vi "WS1050_36 DUT CV Curve SData Ver1.0.vi"(0 "TMN DC\\CAP Data Log File Path":path=path "C:/temp", 1 "Lot#":string="WS1050", 2 "Total Delta C1(pF)":string[](array[string]), 3 "VSA_V1":string[][](array[string]), 4 "Wafer#":string="T7", 5 "File Name":string="Test Data", 6 "Total Delta C2(pF)":string[](array[string]), 7 "error in":errorcluster, 8 "TP/Comment":T1={"Test Program"="Multi Socket", "Comment"="HD_Cycling", "DVA"="", "EFUSE CAL"="", "CP HD/CYC"="", "VDD"="", "Duty Cycle"="", "V_Test(V)"="", "V_VPI(V)"="", "Freq(Hz)"="", "Board#"=""}, 9 "EFuse":string[](array[string])=["NC", "NC", "NC", "NC", "NC", "NC", "NC", "NC", "NC", "NC", "NC", "NC", "NC", "NC", "NC", "NC", "NC", "NC", "NC", "NC", "NC", "NC", "NC", "NC", "NC", "NC", "NC", "NC", "NC", "NC", "NC", "NC", "NC", "NC", "NC", "NC"], 10 "Data Output C3":string[][](table), 11 "Temperature":string="WS1033", 12 "VSA_V2":string[][](array[string]), 13 "VPI C3":string[][](array[string]), 14 "Data Output C1":string[][](table), 15 "VPI C2":string[][](array[string]), 16 "SN":string[](array[string])=["1", "2", "3", "4", "5", "6", "7", "8", "9", "10", "11", "12", "13", "14", "15", "16", "17", "18", "19", "20", "21", "22", "23", "24", "25", "26", "27", "28", "29", "30", "31", "32", "33", "34", "35", "36"], 17 "R/W Status":string[](array[string])=["PASS", "PASS", "PASS", "PASS", "PASS", "PASS", "PASS", "PASS", "PASS", "PASS", "PASS", "PASS", "PASS", "PASS", "PASS", "PASS", "PASS", "PASS", "PASS", "PASS", "PASS", "PASS", "PASS", "PASS", "PASS", "PASS", "PASS", "PASS", "PASS", "PASS", "PASS", "PASS", "PASS", "PASS", "PASS", "PASS"], 18 "Cap Header":string[](array[string]), 20 "HD/Cycles Completed":string="Test Data", 21 "Data Output C2":string[][](table), 23 "VSA_V3":string[][](array[string]), 24 "Current":string[](array[string]), 25 "VPI C1":string[][](array[string]), 26 "Total Delta C3(pF)":string[](array[string])) -> (27 "error out":errorcluster)   [LabVIEW 2012]
panel:
  in  "Bin":string[](array[string])=["NC", "NC", "NC", "NC", "NC", "NC", "NC", "NC", "NC", "NC", "NC", "NC", "NC", "NC", "NC", "NC", "NC", "NC", "NC", "NC", "NC", "NC", "NC", "NC", "NC", "NC", "NC", "NC", "NC", "NC", "NC", "NC", "NC", "NC", "NC", "NC"]
  # "*********** Do Not Remove ***********\nCompany:  WiSpry Inc\n20 Fairbanks Ste 198 Irvine CA 92618\n\nAuthor:  Andy V Tran\nCreated:  09/17/2014\nLabVIEW 2012 Suite\nTP:  Multi-Socket Save Data ver1.0\n*****************************************"
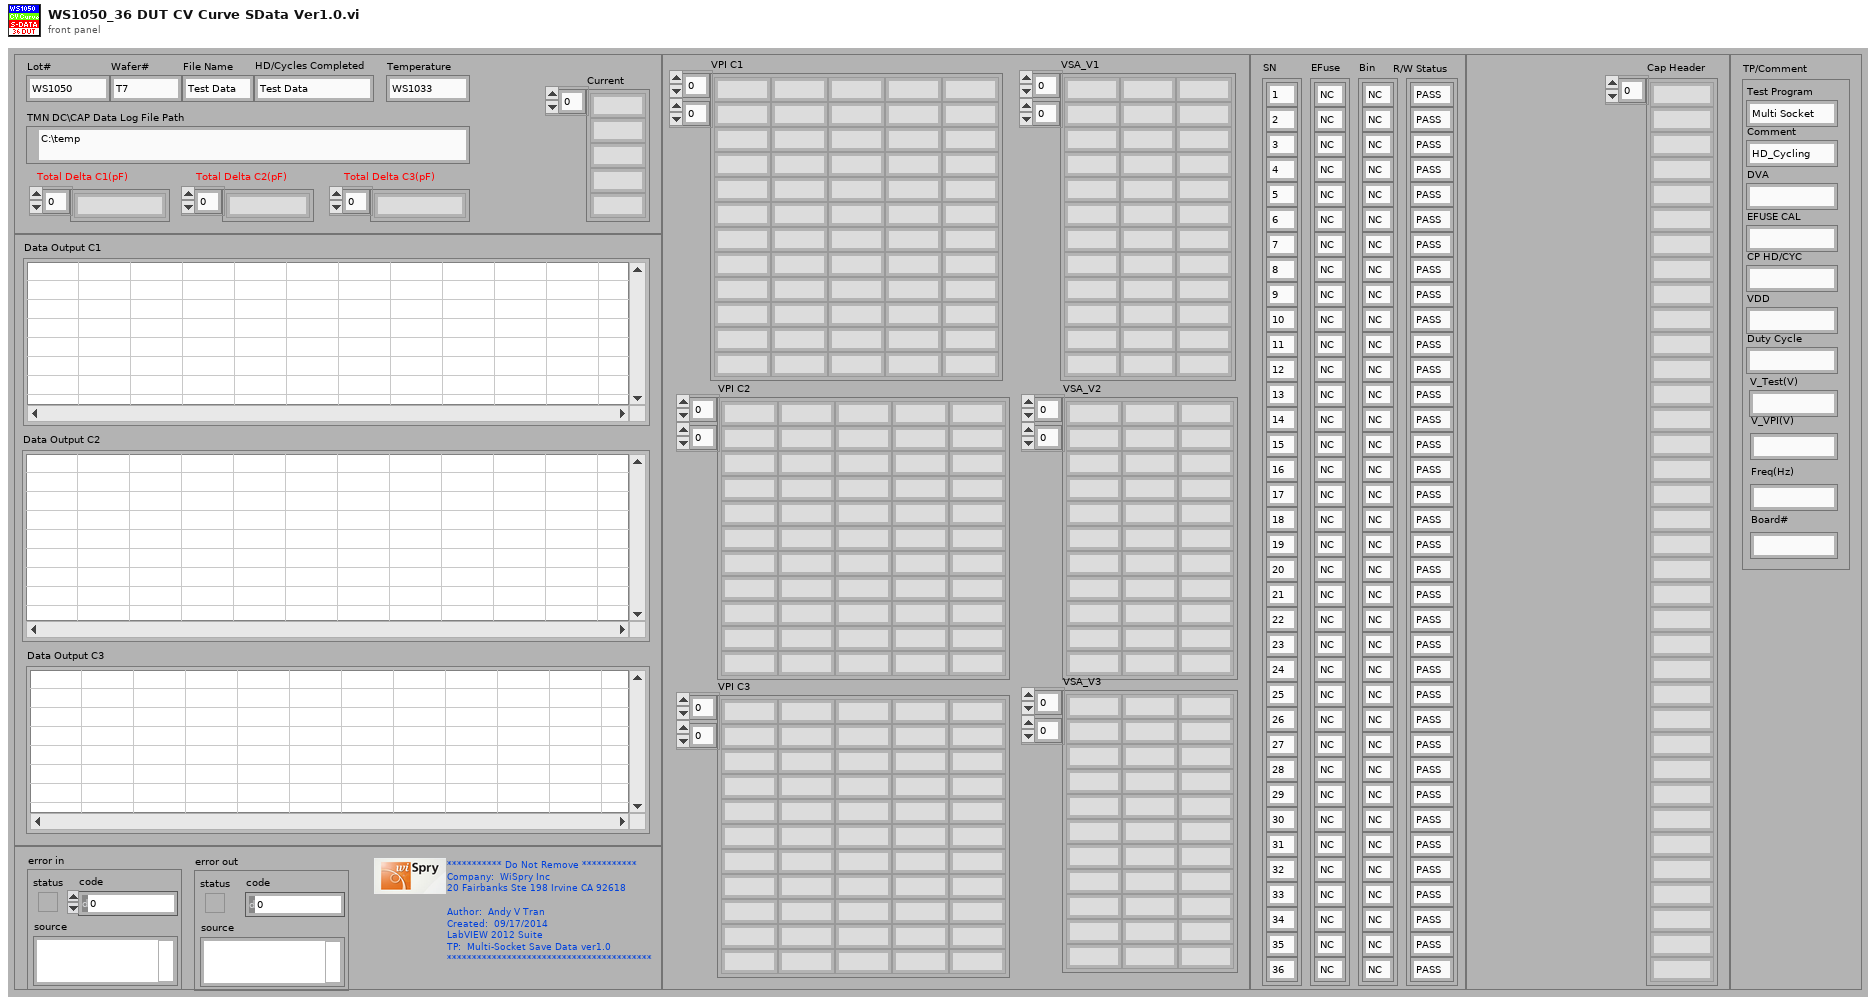
[diagram p1: front panel]
types:
  T1 = cluster{"Test Program":string, "Comment":string, "DVA":string, "EFUSE CAL":string, "CP HD/CYC":string, "VDD":string, "Duty Cycle":string, "V_Test(V)":string, "V_VPI(V)":string, "Freq(Hz)":string, "Board#":string}
  T2 = enum16{"open", "replace", "create", "open or create", "replace or create", "replace or create with confirmation"}
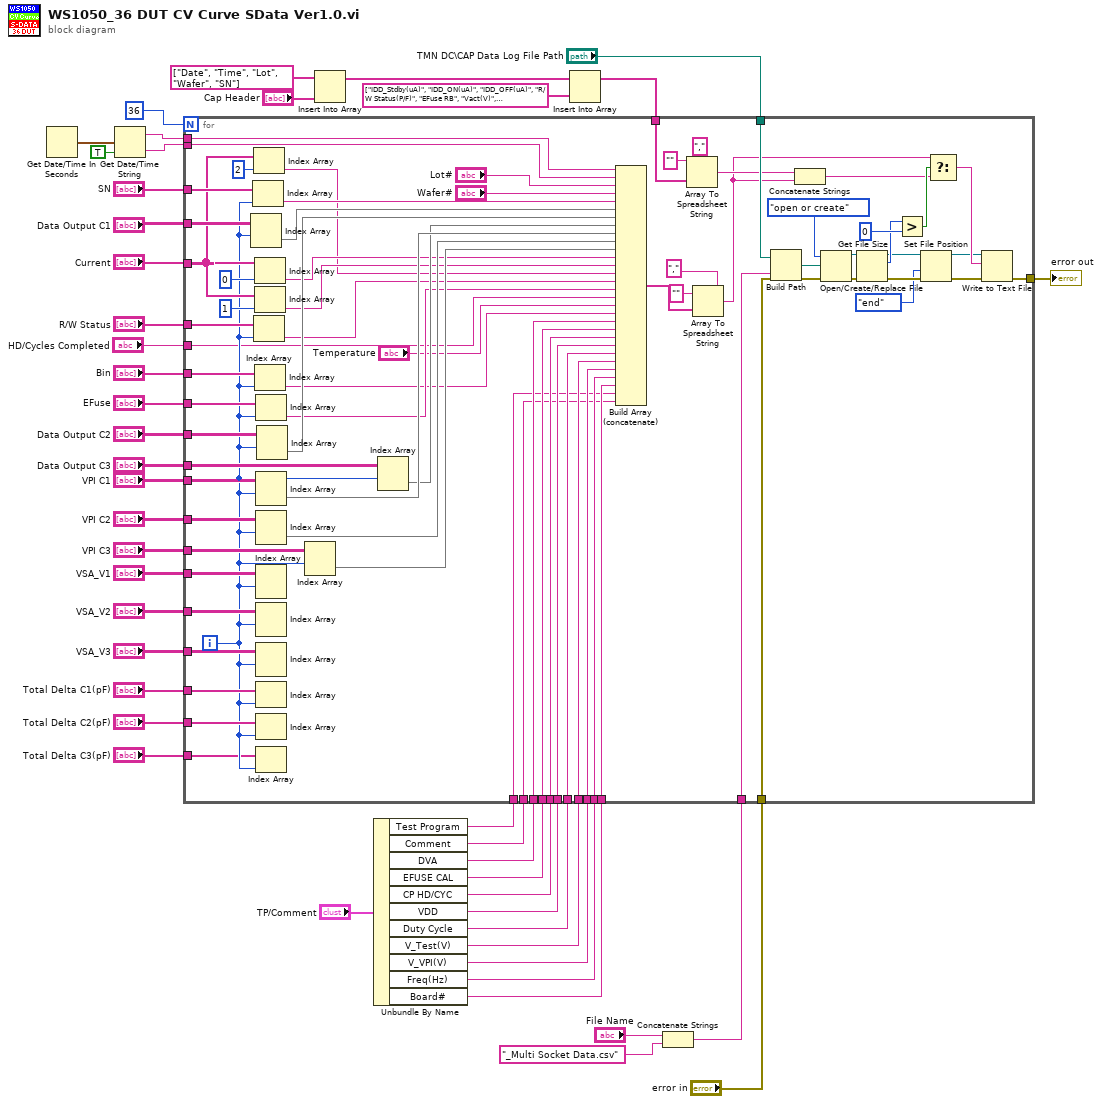
[diagram p0: block diagram]
diagram:
  n1 = Get Date/Time In Seconds() -> (seconds since 1Jan1904=w25:timestamp)
  n2 = Get Date/Time String(seconds (now)=w25, want seconds? (F)=TRUE) -> (date string=w33:string, time string=w34:string)  [unwired: 1 in]
  n3 = Insert Into Array(array=string[] ["Date", "Time", "Lot", "Wafer", "SN"], new element="Cap Header") -> (w12:string[])  [unwired: 1 in]
  n4 = Unbundle By Name("TP/Comment") -> ("Test Program"=w38:string, "Comment"=w37:string, "DVA"=w11:string, "EFUSE CAL"=w10:string, "CP HD/CYC"=w9:string, "VDD"=w8:string, "Duty Cycle"=w7:string, "V_Test(V)"=w6:string, "V_VPI(V)"=w5:string, "Freq(Hz)"=w3:string, "Board#"=w2:string)
  n5 = Insert Into Array(array=w12, new element=string[] ["IDD_Stdby(uA)", "IDD_ON(uA)", "IDD_OFF(uA)", "R/W Status(P/F)", "EFuse RB", "Vact(V)", "Temperature", "Bin", "DVA ON/OFF", "CAL ON/OFF", "CP_Sweep(V)", "VDD", "Duty Cycle(%)", "V_Test(V)", "V_VPI(V)", "Freq(Hz)", "Board", "Test Program", "Comment"]) -> (w16:string[])  [unwired: 1 in]
  n6 = Concatenate Strings("File Name", "_Multi Socket Data.csv" ("string")) -> (w41:string)
  n7 = for {
    N: 36 -> [_]
    tunnel: "TMN DC\\CAP Data Log File Path" -> [w123]
    tunnel: w16 -> [w122]
    tunnel: "error in" -> [w83]
    tunnel: w41 -> [w121]
    tunnel: [w99] -> w40
    tunnel: "SN" -> [w98]
    tunnel: "Current" -> [w90]
    tunnel: w38 -> [w48]
    tunnel: w37 -> [w47]
    tunnel: "Bin" -> [w97]
    tunnel: "R/W Status" -> [w96]
    tunnel: w34 -> [w73]
    tunnel: w33 -> [w72]
    tunnel: "Data Output C1" -> [w95]
    tunnel: "Data Output C2" -> [w94]
    tunnel: "VPI C1" -> [w89]
    tunnel: "VPI C2" -> [w88]
    tunnel: "EFuse" -> [w87]
    tunnel: "VSA_V1" -> [w86]
    tunnel: "VSA_V2" -> [w85]
    tunnel: "VSA_V3" -> [w84]
    tunnel: "VPI C3" -> [w82]
    tunnel: "Data Output C3" -> [w81]
    tunnel: "Total Delta C1(pF)" -> [w71]
    tunnel: "Total Delta C2(pF)" -> [w70]
    tunnel: "Total Delta C3(pF)" -> [w68]
    tunnel: w11 -> [w57]
    tunnel: w10 -> [w56]
    tunnel: w9 -> [w55]
    tunnel: w8 -> [w54]
    tunnel: w7 -> [w53]
    tunnel: w6 -> [w52]
    tunnel: w5 -> [w51]
    tunnel: "HD/Cycles Completed" -> [w60]
    tunnel: w3 -> [w50]
    tunnel: w2 -> [w49]
    i -> [w69]
    n8 = Index Array(array=w95, index (row)=w69) -> (element=w75:string[])  [unwired: 1 in]
    n9 = Index Array(array=w98, index=w69) -> (element=w74:string)
    n10 = Index Array(array=w90, index=2) -> (element=w63:string)
    n11 = Index Array(array=w96, index=w69) -> (element=w62:string)
    n12 = Index Array(array=w90, index=0) -> (element=w65:string)
    n13 = Index Array(array=w90, index=1) -> (element=w64:string)
    n14 = Index Array(array=w97, index=w69) -> (element=w58:string)
    n15 = Index Array(array=w87, index=w69) -> (element=w61:string)
    n16 = Index Array(array=w89, index (row)=w69) -> (element=w78:string[])  [unwired: 1 in]
    n17 = Index Array(array=w88, index (row)=w69) -> (element=w79:string[])  [unwired: 1 in]
    n18 = Index Array(array=w86, index (row)=w69) -> ()  [unwired: 1 in, 1 out]
    n19 = Index Array(array=w85, index (row)=w69) -> ()  [unwired: 1 in, 1 out]
    n20 = Index Array(array=w84, index (row)=w69) -> ()  [unwired: 1 in, 1 out]
    n21 = Index Array(array=w71, index=w69) -> ()  [unwired: 1 out]
    n22 = Index Array(array=w70, index=w69) -> ()  [unwired: 1 out]
    n23 = Index Array(array=w68, index=w69) -> ()  [unwired: 1 out]
    n24 = Index Array(array=w94, index (row)=w69) -> (element=w76:string[])  [unwired: 1 in]
    n25 = Index Array(array=w82, index (row)=w69) -> (element=w80:string[])  [unwired: 1 in]
    n26 = Index Array(array=w81, index (row)=w69) -> (element=w77:string[])  [unwired: 1 in]
    n27 = Build Array (concatenate)(w72, w73, "Lot#", "Wafer#", w74, w75, w76, w77, w78, w79, w80, w65, w64, w63, w62, w61, w60, "Temperature", w58, w57, w56, w55, w54, w53, w52, w51, w50, w49, w48, w47) -> (w100:string[])
    n28 = Array To Spreadsheet String(delimiter (Tab)=",", array=w122, 3:"" ("format string")) -> (spreadsheet string=w103:string)
    n29 = Array To Spreadsheet String(delimiter (Tab)=",", array=w100, 3:"" ("format string")) -> (spreadsheet string=w101:string)
    n30 = Build Path(base path=w123, name or relative path=w121) -> (appended path=w115:path)
    n31 = Concatenate Strings(w103, w101) -> (w102:string)
    n32 = Open/Create/Replace File(file path (use dialog)=w115, error in=w83, operation (0:open)=T2."open or create") -> (refnum out=w113:refnum<file>, error out=w116:errorcluster)  [unwired: 4 out]
    n33 = Get File Size(file=w113, error in=w116) -> (refnum out=w108:refnum<file>, size (in bytes)=w112:i64, 0:w110:errorcluster)
    n34 = Greater?(x=w112, y=i64 0) -> (0:w117:bool)
    n35 = Set File Position(refnum=w108, from (0:start)=enum16{"start", "end", "current"}."end", error in=w110) -> (refnum out=w107:refnum<file>, error out=w109:errorcluster)  [unwired: 1 out]
    n36 = Select(t=w101, s=w117, f=w102) -> (s? t:f=w114:string)
    n37 = Write to Text File(file (use dialog)=w107, text=w114, error in=w109) -> (error out=w99:errorcluster)  [unwired: 3 out]
  }
  "error out" <- w40
